vi "Area of Square.vi"() -> ()   [LabVIEW 2011]
panel:
  in  "stop":bool
  out "Area":dbl=3.141592653589793 format="%#_8g"
  in  "Width":dbl(slide) scale=0.0..10.0
  in  "Height":dbl(slide) scale=0.0..10.0
  out "Hello Pi":dbl=3.141592653589793 format="%#_8g"
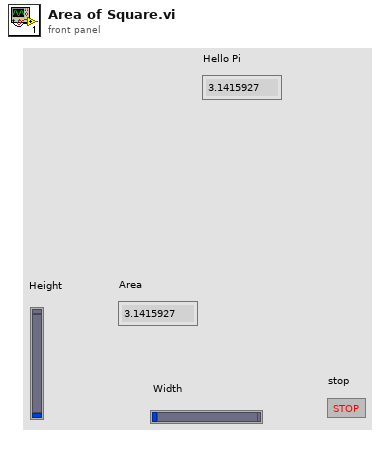
[diagram p1: front panel]
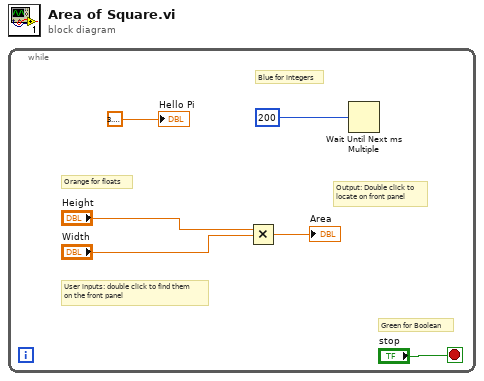
[diagram p0: block diagram]
diagram:
  n1 = while {
    stop <- "stop" stop-if-true
    # "Output: Double click to \nlocate on front panel"
    # "Green for Boolean"
    # "Orange for floats"
    # "Blue for integers"
    # "User inputs: double click to find them\non the front panel"
    n2 = Multiply(x="Height", y="Width") -> (x*y=→"Area":dbl)
    n3 = Wait Until Next ms Multiple(millisecond multiple=u32 200 ("millisecond timer value")) -> ()  [unwired: 1 out]
    "Hello Pi" <- 3.141592653589793
  }
